vi "Load Image.vi"(8 "error in":errorcluster, 11 "File":string="c:\\temp\\hello.bmp") -> (0 "error out":errorcluster, 3 "Surface Pointer":u32 format="%.0x")   [LabVIEW 2014, in "LibSDL2.lvlib"]
uses:
  LibSDL2.lvlib
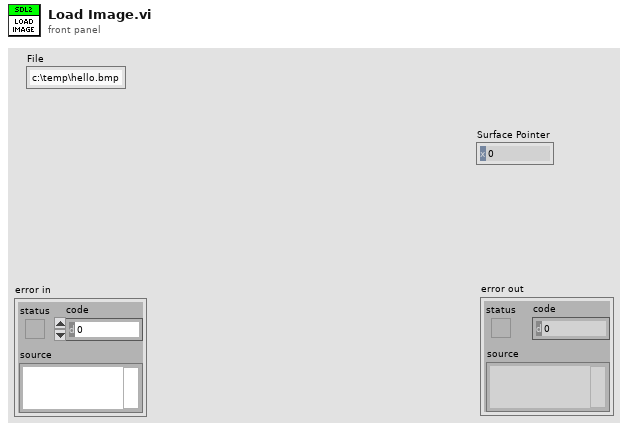
[diagram p1: front panel]
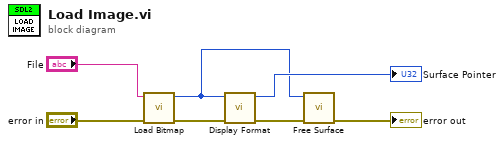
[diagram p0: block diagram]
diagram:
  n1 = call "Load Bitmap.vi"("error in"="error in", "File"="File") -> ("error out"=w5:errorcluster, "Surface Pointer"=w2:u32)  [unwired: 8 in]
  n2 = call "Display Format.vi"("error in"=w5, "Surface Pointer"=w2) -> ("error out"=w4:errorcluster, "Surface Pointer"=→"Surface Pointer":u32)  [unwired: 8 in]
  n3 = call "Free Surface.vi"("error in"=w4, "Surface Pointer"=w2) -> ("error out"=→"error out":errorcluster)  [unwired: 9 in]
